vi "Set Channel Color.vi"(8 "error in (no error)":errorcluster, 9 "Channel Color":u32(colorbox)=6618880, 10 "Channel":u16(ring) items=["A1"=0, "A2"=1, "A3"=2, "A4"=3, "A5"=4, "A6"=5, "A7"=6, "A8"=7, "A9"=8, "A10"=9, "K1"=200, "K2"=201, "K3"=202, "K4"=203, "FA1"=204, "FA2"=205, "FA3"=206, "FA4"=207], 11 "VISA resource name":refnum<visa-resource-name>) -> (0 "error out":errorcluster, 3 "VISA resource name out":refnum<visa-resource-name>)   [LabVIEW 2017, in "Sefram DAS220.lvlib"]
doc: "Set the channel color in the recorder"
uses:
  <instrlib>/Sefram DAS220/Sefram DAS220.lvlib
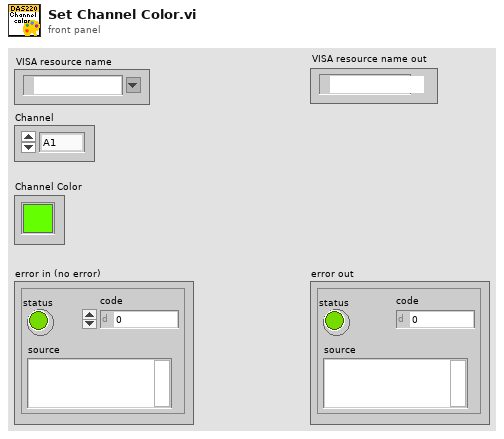
[diagram p1: front panel]
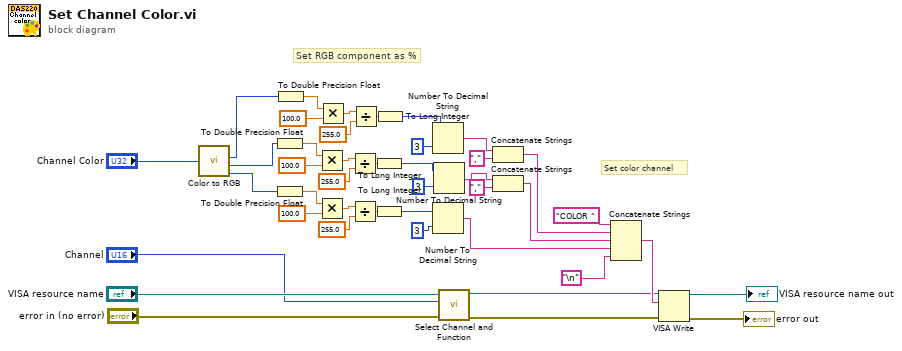
[diagram p0: block diagram]
diagram:
  # "Set RGB component as %"
  # "Set color channel"
  n1 = call <vilib>:"Color to RGB.vi"("Color"="Channel Color") -> ("R"=w11:u8, "G"=w17:u8, "B"=w26:u8)  [unwired: 1 out]
  n2 = To Double Precision Float(number=w17) -> (double precision float=w19:dbl)
  n3 = To Double Precision Float(number=w26) -> (double precision float=w25:dbl)
  n4 = To Double Precision Float(number=w11) -> (double precision float=w13:dbl)
  n5 = Multiply(x=w19, y=100.0) -> (x*y=w21:dbl)
  n6 = Multiply(x=w25, y=100.0) -> (x*y=w28:dbl)
  n7 = Multiply(x=w13, y=100.0) -> (x*y=w15:dbl)
  n8 = Divide(x=w21, y=255.0) -> (x/y=w18:dbl)
  n9 = Divide(x=w28, y=255.0) -> (x/y=w24:dbl)
  n10 = Divide(x=w15, y=255.0) -> (x/y=w12:dbl)
  n11 = To Long Integer(number=w18) -> (32bit integer=w9:i32)
  n12 = To Long Integer(number=w24) -> (32bit integer=w23:i32)
  n13 = To Long Integer(number=w12) -> (32bit integer=w10:i32)
  n14 = Number To Decimal String(number=w10, width (-)=i16 3) -> (decimal integer string=w36:string)
  n15 = Number To Decimal String(number=w23, width (-)=i16 3) -> (decimal integer string=w30:string)
  n16 = Number To Decimal String(number=w9, width (-)=i16 3) -> (decimal integer string=w32:string)
  n17 = call <instrlib>:"Select Channel and Function.vi"("error in (no error)"="error in (no error)", "Channel"="Channel", "VISA resource name"="VISA resource name") -> ("error out"=w3:errorcluster, "VISA resource name out"=w5:refnum<visa-resource-name>)  [unwired: 7 in]
  n18 = Concatenate Strings(w36, "," ("string")) -> (w34:string)
  n19 = Concatenate Strings(w32, "," ("string")) -> (w31:string)
  n20 = Concatenate Strings("COLOR " ("string"), w34, w31, w30, "\n") -> (w42:string)
  n21 = VISA Write(VISA resource name=w5, write buffer=w42, error in (no error)=w3) -> (VISA resource name out=→"VISA resource name out":refnum<visa-resource-name>, error out=→"error out":errorcluster)  [unwired: 1 out]
